vi "Apply Theme To TitleBar-Title.vi"(8 "Error In":errorcluster, 9 "Override Root With (Empty)":string, 10 "Title Ref":refnum<vi>, 11 "Generic Theme in":refnum<class "Generic Theme.lvclass">) -> (0 "Error Out":errorcluster, 3 "Generic Theme out":refnum<class "Generic Theme.lvclass">)   [LabVIEW 2021, in "Appearance Actor.lvlib" / "Generic Theme.lvclass"]
uses:
  Generic Theme.lvclass
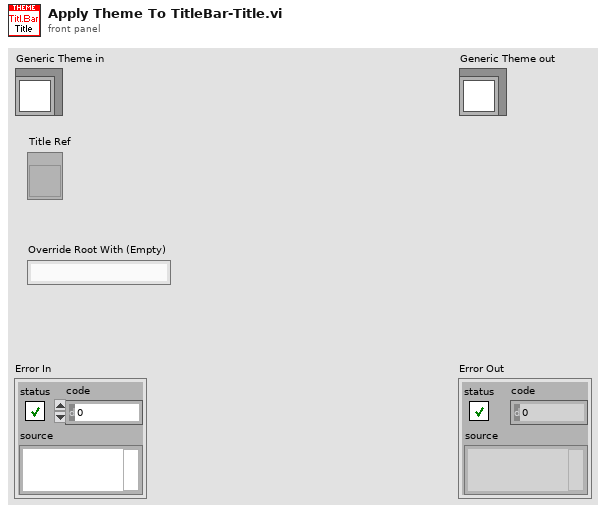
[diagram p1: front panel]
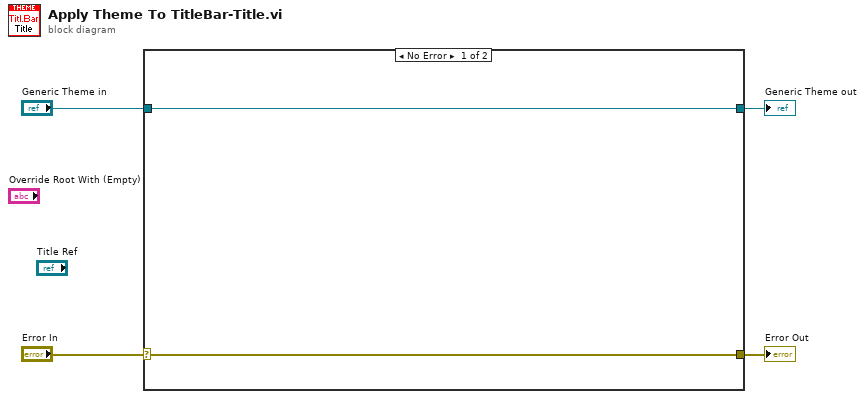
[diagram p0: block diagram]
diagram:
  n1 = case shown="No Error" "Error In" {
    selector: "Error In" -> [w5 w8]
    tunnel: [w5 w8] -> w3
    tunnel: [w6 w7] -> w1
    tunnel: "Generic Theme in" -> [w6 w7]
    frame No Error {
    }
    frame Error {
    }
  }
  "Error Out" <- w3
  "Generic Theme out" <- w1
